vi "SetMotor.vi"(8 "error in (no error)":errorcluster, 10 "index(0..3)":i32, 11 "Motorshield in":refnum<class "Motorshield.lvclass">) -> (0 "error out":errorcluster, 1 "Motorinfo":T1, 2 "index":i32, 3 "Motorshield out":refnum<class "Motorshield.lvclass">)   [LabVIEW 2022 SP3, in "Motorshield.lvlib" / "Motorshield.lvclass"]
uses:
  Motorshield.lvclass
  DCMotor/MotorInfo.ctl
  Motorshield.lvclass/Motorshield.ctl
  DCMotor/DCMotor.lvclass
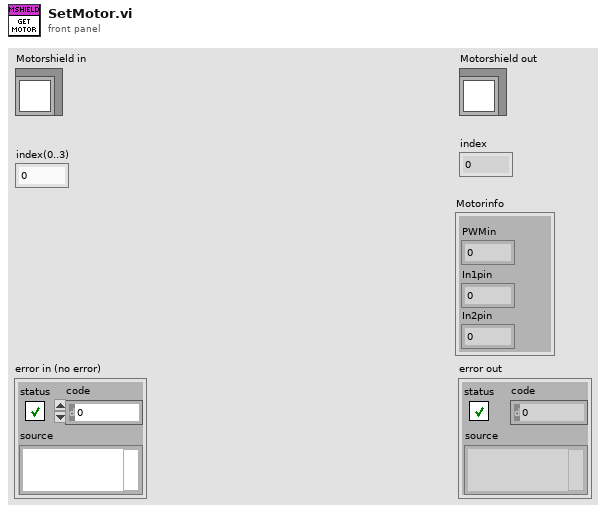
[diagram p1: front panel]
types:
  T1 = typedef "Motorshield.lvlib/DCMotor.lvclass/MotorInfo.ctl" = cluster{"PWMin":u8, "In1pin":u8, "In2pin":u8}
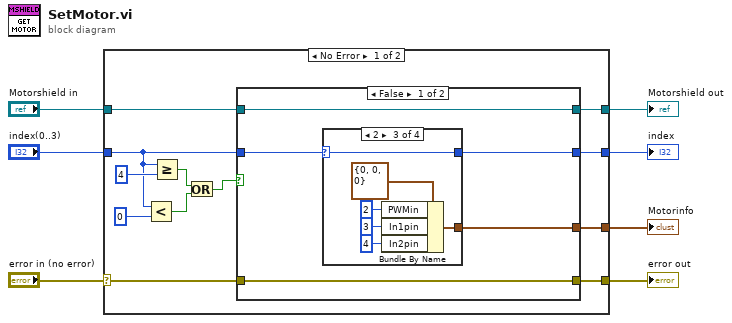
[diagram p0: block diagram]
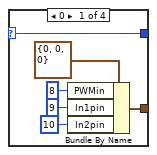
[diagram p2: hidden frame]
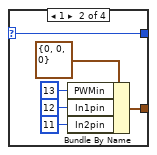
[diagram p3: hidden frame]
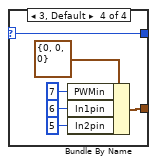
[diagram p4: hidden frame]
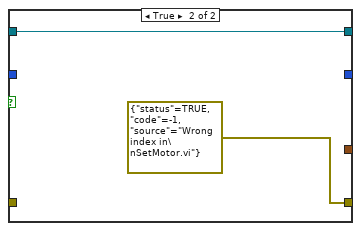
[diagram p5: hidden frame]
diagram:
  n1 = case shown="No Error" "error in (no error)" {
    selector: "error in (no error)" -> [w17 w51]
    tunnel: [w15 w52] -> w5
    tunnel: "Motorshield in" -> [w19 w52]
    tunnel: "index(0..3)" -> [w12 _]
    tunnel: [w16 w51] -> w3
    tunnel: [w9 _] -> w2
    tunnel: [w8 _] -> w1
    frame No Error {
      n2 = Less?(x=w12, y=0) -> (x < y?=w10:bool)
      n3 = Greater Or Equal?(x=w12, y=4) -> (x >= y?=w13:bool)
      n4 = Or(x=w13, y=w10) -> (x .or. y?=w14:bool)
      n5 = case shown="False" w14 {
        tunnel: w19 -> [w22 w50]
        tunnel: w12 -> [w24 _]
        tunnel: w17 -> [w23 _]
        tunnel: [w23 errorcluster {"status"=TRUE, "code"=-1, "source"="Wrong index in\nSetMotor.vi"} ("error IO")] -> w16
        tunnel: [w22 w50] -> w15
        tunnel: [w20 _] -> w9
        tunnel: [w21 _] -> w8
        frame False {
          n6 = case shown="2" w24 {
            selector: w24 -> [w26 w32 w38 w44]
            tunnel: [w26 w32 w38 w44] -> w20
            tunnel: [w25 w31 w37 w43] -> w21
            frame 0 {
              n7 = Bundle By Name(cluster=T1 {"PWMin"=0, "In1pin"=0, "In2pin"=0} ("Motorinfo"), "PWMin"=u8 8, "In1pin"=u8 9, "In2pin"=u8 10) -> (w25:T1)
            }
            frame 1 {
              n8 = Bundle By Name(cluster=T1 {"PWMin"=0, "In1pin"=0, "In2pin"=0} ("Motorinfo"), "PWMin"=u8 13, "In1pin"=u8 12, "In2pin"=u8 11) -> (w31:T1)
            }
            frame 2 {
              n9 = Bundle By Name(cluster=T1 {"PWMin"=0, "In1pin"=0, "In2pin"=0} ("Motorinfo"), "PWMin"=u8 2, "In1pin"=u8 3, "In2pin"=u8 4) -> (w37:T1)
            }
            frame 3, Default {
              n10 = Bundle By Name(cluster=T1 {"PWMin"=0, "In1pin"=0, "In2pin"=0} ("Motorinfo"), "PWMin"=u8 7, "In1pin"=u8 6, "In2pin"=u8 5) -> (w43:T1)
            }
          }
        }
        frame True {
        }
      }
    }
    frame Error {
    }
  }
  "error out" <- w3
  "Motorshield out" <- w5
  "index" <- w2
  "Motorinfo" <- w1
